vi "SampleGetIDSingle_8742.vi"() -> ()   [LabVIEW 2009]
panel:
  out "Identification":string
  out "error out":errorcluster
  out "DeviceKey Out":string
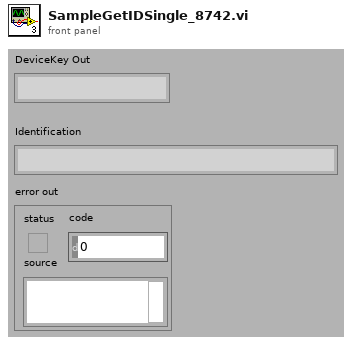
[diagram p1: front panel]
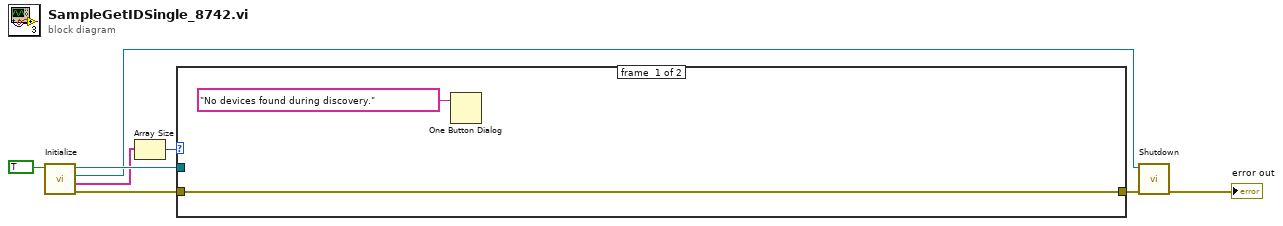
[diagram p0: block diagram]
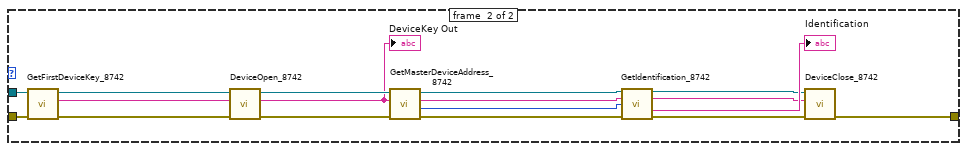
[diagram p2: hidden frame]
diagram:
  n1 = call "Initialize.vi"("logging"=TRUE) -> ("error out"=w4:errorcluster, "DeviceKey List"=w2:string[], "DeviceIOLib Out"=w3:refnum<k24>, "CmdLib Out"=w5:refnum<k24>)  [unwired: 3 in]
  n2 = Array Size(array=w2) -> (size(s)=w1:i32)
  n3 = case shown="1, Default" w1 {
    tunnel: [w10 w18] -> w6
    tunnel: w5 -> [_ w22]
    tunnel: w4 -> [w10 w21]
    frame #0 {
      n4 = One Button Dialog(message="No devices found during discovery.") -> ()  [unwired: 1 in, 1 out]
    }
    frame #1 {
      n5 = call "GetFirstDeviceKey_8742.vi"("error in"=w21, "CmdLib In"=w22) -> ("error out"=w16:errorcluster, "DeviceKey Out"=w12:string, "CmdLib Out"=w14:refnum<k24>)  [unwired: 3 in]
      n6 = call "DeviceOpen_8742.vi"("error in (no error)"=w16, "DeviceKey In"=w12, "CmdLib In"=w14) -> ("error out"=w15:errorcluster, "DeviceKey Out"=w11:string, "CmdLib Out"=w13:refnum<k24>)  [unwired: 2 in]
      "DeviceKey Out" <- w11
      n7 = call "GetMasterDeviceAddress_8742.vi"("error in (no error)"=w15, "DeviceKey In"=w11, "CmdLib In"=w13) -> ("error out"=w26:errorcluster, "Device Address"=w23:i32, "DeviceKey Out"=w24:string, "CmdLib Out"=w25:refnum<k24>)  [unwired: 1 in]
      n8 = call "GetIdentification_8742.vi"("CmdLib In"=w25, "DeviceKey In"=w24, "Device Address In"=w23, "error in (no error)"=w26) -> ("CmdLib Out"=w20:refnum<k24>, "DeviceKey Out"=w17:string, "Identification"=→"Identification":string, "error out"=w19:errorcluster)  [unwired: 7 in, 1 out]
      n9 = call "DeviceClose_8742.vi"("error in (no error)"=w19, "DeviceKey In"=w17, "CmdLib In"=w20) -> ("error out"=w18:errorcluster)  [unwired: 2 in, 2 out]
    }
  }
  n10 = call "Shutdown.vi"("error in (no error)"=w6, "DeviceIOLib In"=w3) -> ("error out"=→"error out":errorcluster)  [unwired: 5 in]
